vi "FTW-ActorTemplate.vi"(0 "FTW Actor Instance Configuration":string="{\n  \"Identity\": \"ActorName\",\n  \"InboxAddress\": \"tcp://127.0.0.1:*\",\n  \"DebugEnableInboxLogging\": false,\n  \"DebugEnableJobLogging\": false,\n  \"DebugShowPanel\": false\n}", 11 "ErrorIn":errorcluster) -> (15 "Error":errorcluster)   [LabVIEW 2014]
uses:
  src/core/actor/instance/FTW-Actor-Instance.lvclass
  src/core/actor/instance/FTW-Actor-Instance.lvclass/FTW-Actor-Instance.ctl
  src/core/actor/scheduler/FTW-Scheduler-GetNextJob.vi
  src/core/actor/scheduler/FTW-Scheduler-Current.vi
  src/core/actor/request/FTW-Request.lvclass
panel:
  # "Inputs"
  # "Outputs"
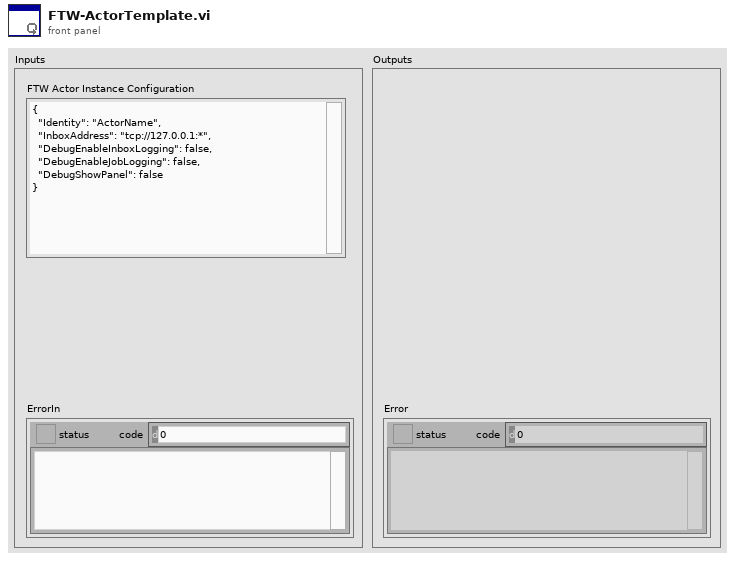
[diagram p1: front panel]
types:
  T1 = cluster{"Incoming Requests":refnum<event-registration>, "Additional Registration Types":refnum<event-registration>}
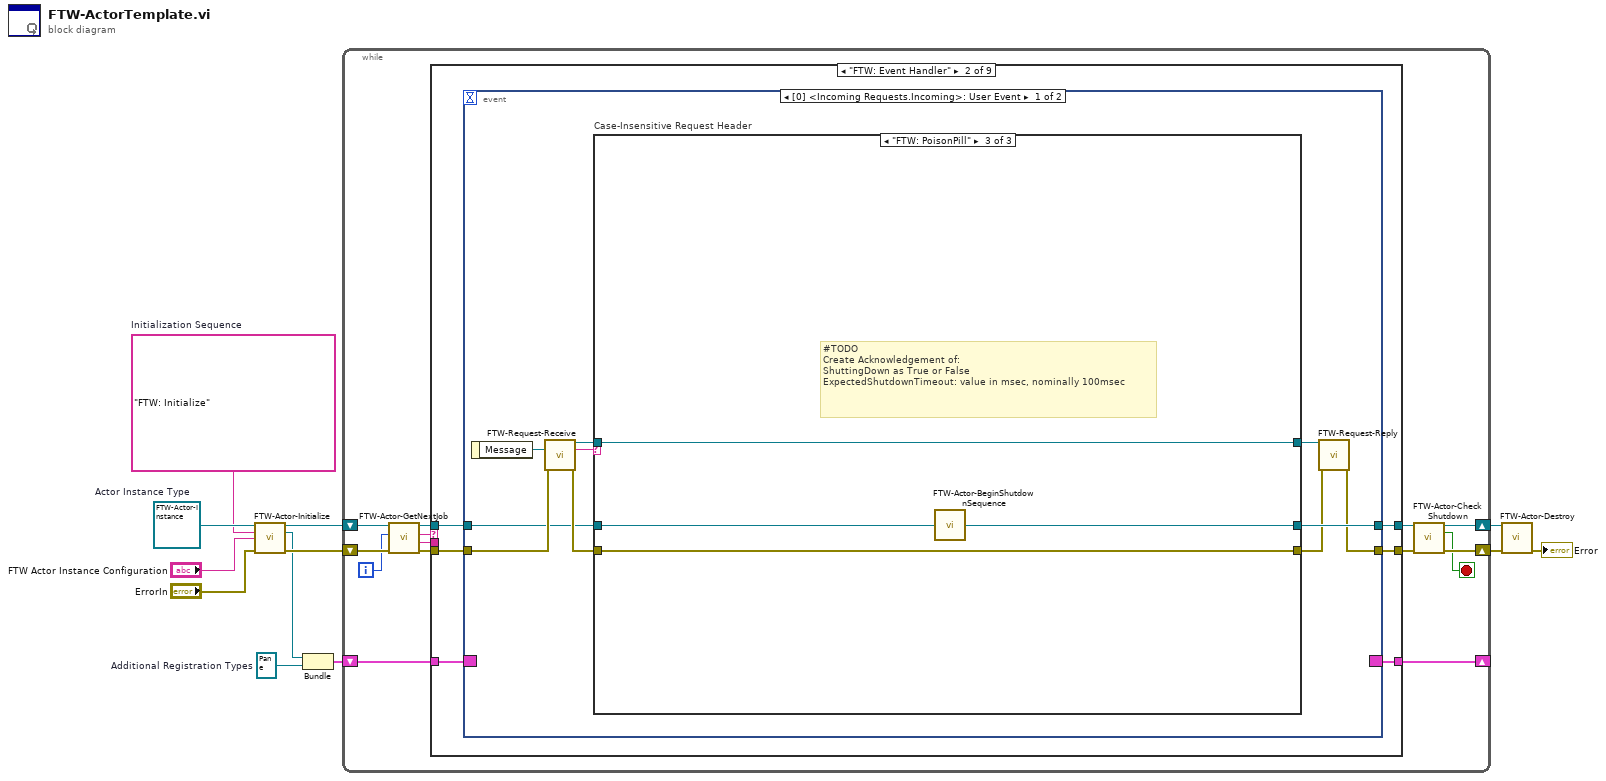
[diagram p0: block diagram]
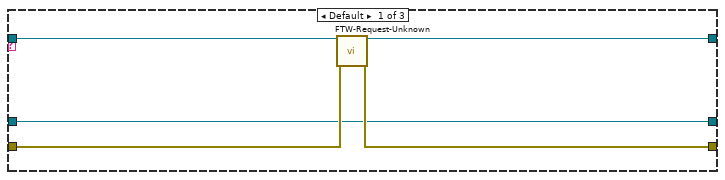
[diagram p3: hidden frame]
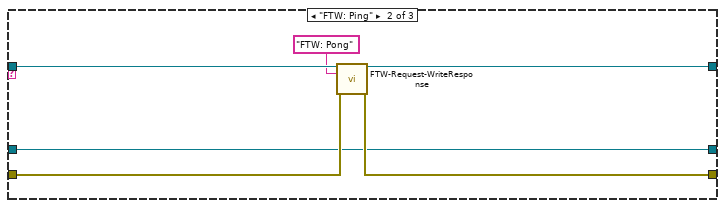
[diagram p4: hidden frame]
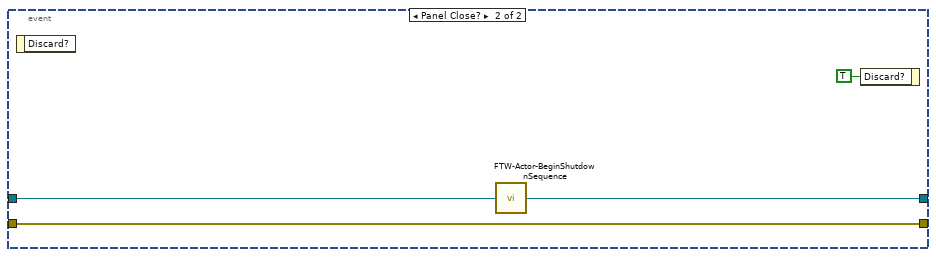
[diagram p5: hidden frame]
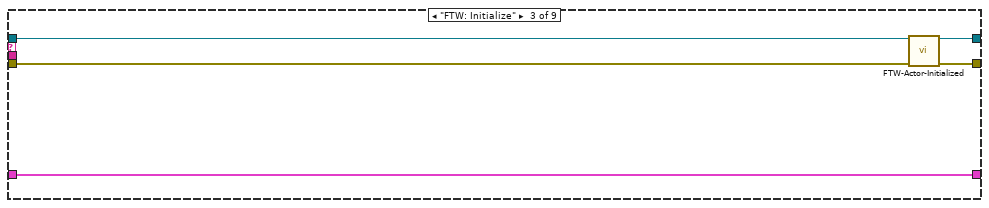
[diagram p6: hidden frame]
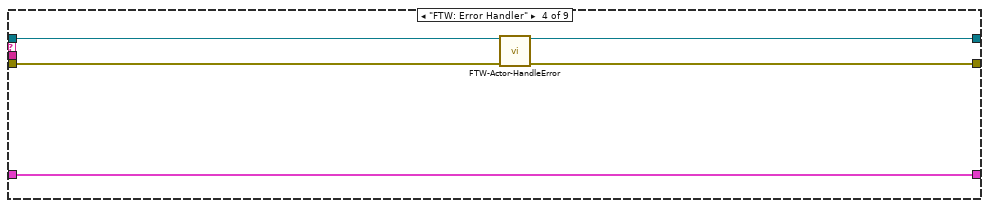
[diagram p7: hidden frame]
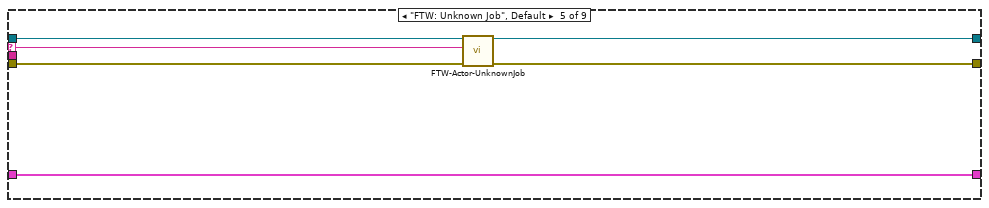
[diagram p8: hidden frame]
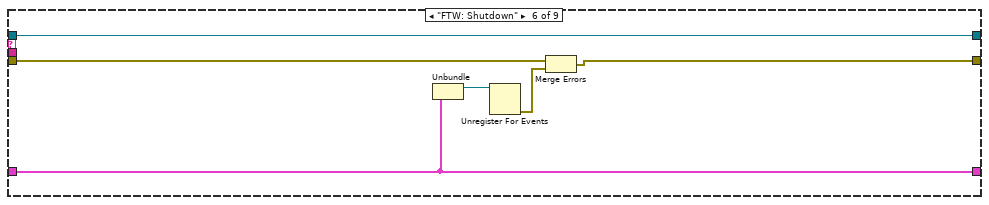
[diagram p9: hidden frame]
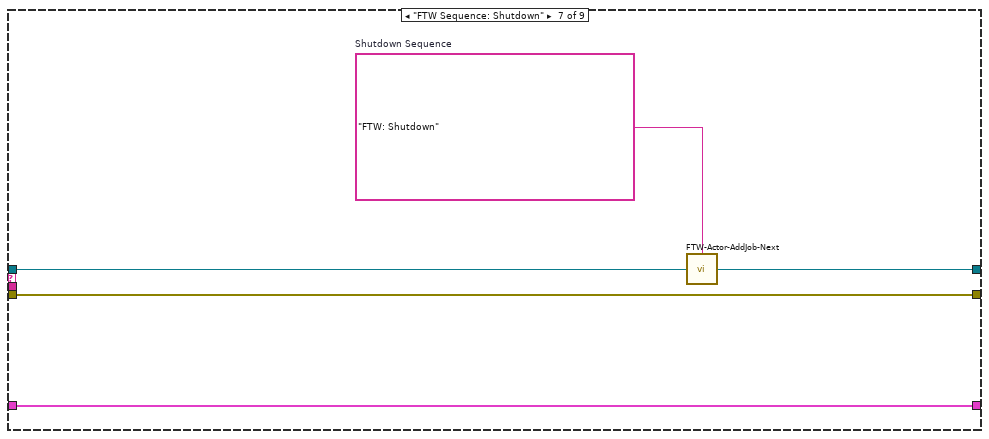
[diagram p10: hidden frame]
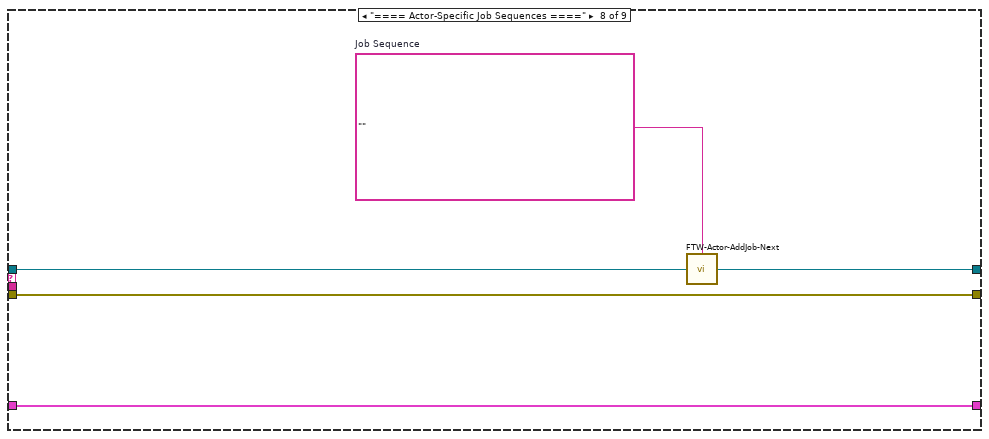
[diagram p11: hidden frame]
diagram:
  w4 = refnum<event-registration> refnum  # Additional Registration Types
  w7 = refnum<class "FTW-Actor-Instance.lvclass"> refnum  # Actor Instance Type
  w6 = "FTW: Initialize"  # Initialization Sequence
  n1 = call "FTW-Actor-Initialize.vi"("FTW Actor Instance Type"=w7, "Initialization Job Sequence"=w6, "Actor Instance Configuration"="FTW Actor Instance Configuration", "error in"="ErrorIn") -> ("FTW Actor Instance"=w12:refnum<class "FTW-Actor-Instance.lvclass">, "Incoming Requests"=w1:refnum<event-registration>, "error out"=w8:errorcluster)  [unwired: 9 in]
  n2 = Bundle("Incoming Requests"=w1, "Additional Registration Types"=w4) -> (w3:T1)  [unwired: 1 in]
  n3 = while {
    shift-right: [w16] -> w10
    shift-left: w8 -> [w23]
    shift-right: [w13] -> _
    shift-left: w3 -> [w26]
    shift-right: [w18] -> w11
    shift-left: w12 -> [w25]
    i -> [w14]
    stop <- w15 stop-if-true
    n4 = call "FTW-Actor-GetNextJob.vi"("error in"=w23, "Jobs Performed"=w14, "FTW Actor Instance"=w25) -> ("error out"=w22:errorcluster, "Job Data"=w20:string, "Job Name"=w21:string, "FTW Actor Instance out"=w24:refnum<class "FTW-Actor-Instance.lvclass">)  [unwired: 5 in]
    n5 = case shown="\"FTW: Event Handler\"" w21 {
      selector: w21 -> [_ _ _ _ w75 _ _ _ _]
      tunnel: [w28 w35 w65 w70 w78 w83 w90 w95 w99] -> w17
      tunnel: w22 -> [w28 w34 w68 w72 w79 w84 w90 w95 w99]
      tunnel: w26 -> [w29 w30 w69 w74 w80 w86 w91 w96 w98]
      tunnel: [w29 w33 w69 w74 w80 w86 w91 w96 w98] -> w13
      tunnel: w20 -> [_ _ _ _ _ _ _ _ _]
      tunnel: [w27 w32 w66 w71 w76 w81 w88 w93 w97] -> w19
      tunnel: w24 -> [w27 w31 w67 w73 w77 w81 w89 w94 w97]
      frame "==== Featherweight Framework Jobs ====" {
      }
      frame "FTW: Event Handler" {
        n6 = event shown="[0] <Incoming Requests.Incoming>: User Event" {
          selector: w30 -> [_ _]
          dyn-events: [_ _] -> w33
          timeout: _ -> [_ _]
          tunnel: [w39 w63] -> w35
          tunnel: w34 -> [w44 w63]
          tunnel: [w43 w61] -> w32
          tunnel: w31 -> [w42 w62]
          event User Event {
            n7 = event-data() -> ("Message"=w36:refnum<class "FTW-Message.lvclass">)  [unwired: 1 in]
            n8 = call "FTW-Request-Receive.vi"("Message"=w36, "error in"=w44) -> ("Initialized Request"=w40:refnum<class "FTW-Request.lvclass">, "Request Header"=w41:string, "error out"=w45:errorcluster)  [unwired: 11 in]
            n9 = case "Case-Insensitive Request Header" shown="\"FTW: PoisonPill\"" w41 {
              tunnel: [w49 w54 w57] -> w38
              tunnel: w45 -> [w50 w55 w57]
              tunnel: [w47 w52 w60] -> w43
              tunnel: w42 -> [w47 w52 w59]
              tunnel: w40 -> [w48 w56 w58]
              tunnel: [w46 w51 w58] -> w37
              frame Default {
                n10 = call "FTW-Request-Unknown.vi"("FTW Incoming Request"=w48, "error in"=w50) -> ("FTW Incoming Request out"=w46:refnum<class "FTW-Request.lvclass">, "error out"=w49:errorcluster)  [unwired: 12 in]
              }
              frame "FTW: Ping" {
                n11 = call "FTW-Request-WriteResponse.vi"("FTW Incoming Request"=w56, "Response Body"="FTW: Pong" ("Response Header"), "error in"=w55) -> ("FTW Incoming Request out"=w51:refnum<class "FTW-Request.lvclass">, "error out"=w54:errorcluster)  [unwired: 11 in]
              }
              frame "FTW: PoisonPill" {
                # "#TODO\nCreate Acknowledgement of:\nShuttingDown as True or False\nExpectedShutdownTimeout: value in msec, nominally 100msec"
                n12 = call "FTW-Actor-BeginShutdownSequence.vi"("FTW Actor Instance"=w59) -> ("FTW Actor Instance out"=w60:refnum<class "FTW-Actor-Instance.lvclass">)  [unwired: 3 in]
              }
            }
            n13 = call "FTW-Request-Reply.vi"("FTW Incoming Request"=w37, "error in"=w38) -> ("error out"=w39:errorcluster)  [unwired: 12 in, 1 out]
          }
          event Panel Close? {
            n14 = event-data() -> ()  [unwired: 1 in, 1 out]
            n15 = call "FTW-Actor-BeginShutdownSequence.vi"("FTW Actor Instance"=w62) -> ("FTW Actor Instance out"=w61:refnum<class "FTW-Actor-Instance.lvclass">)  [unwired: 3 in]
            n16 = event-data("Discard?"=TRUE) -> ()  [unwired: 1 in, 1 out]
          }
        }
      }
      frame "FTW: Initialize" {
        n17 = call-dynamic "FTW-Actor-Initialized.vi"("FTW Actor Instance"=w67, "error in"=w68) -> ("FTW Actor Instance out"=w66:refnum<class "FTW-Actor-Instance.lvclass">, "error out"=w65:errorcluster)  [unwired: 11 in, 1 out]
      }
      frame "FTW: Error Handler" {
        n18 = call-dynamic "FTW-Actor-HandleError.vi"("FTW Actor Instance"=w73, "error in"=w72) -> ("FTW Actor Instance out"=w71:refnum<class "FTW-Actor-Instance.lvclass">, "error out"=w70:errorcluster)  [unwired: 11 in, 1 out]
      }
      frame "FTW: Unknown Job", Default {
        n19 = call-dynamic "FTW-Actor-UnknownJob.vi"("FTW Actor Instance"=w77, "Unknown Job"=w75, "error in"=w79) -> ("FTW Actor Instance out"=w76:refnum<class "FTW-Actor-Instance.lvclass">, "error out"=w78:errorcluster)  [unwired: 11 in]
      }
      frame "FTW: Shutdown" {
        n20 = Unbundle(w86) -> ("Incoming Requests"=w85:refnum<event-registration>)  [unwired: 1 out]
        n21 = Unregister For Events(event registration refnum=w85) -> (error out=w82:errorcluster)  [unwired: 1 in]
        n22 = Merge Errors(w84, w82) -> (w83:errorcluster)
      }
      frame "FTW Sequence: Shutdown" {
        w87 = "FTW: Shutdown"  # Shutdown Sequence
        n23 = call "FTW-Actor-AddJob-Next.vi"("Add Next in Job Queue"=w87, "FTW Actor Instance"=w89) -> ("FTW Actor Instance out"=w88:refnum<class "FTW-Actor-Instance.lvclass">)  [unwired: 2 in]
      }
      frame "==== Actor-Specific Job Sequences ====" {
        w92 = ""  # Job Sequence
        n24 = call "FTW-Actor-AddJob-Next.vi"("Add Next in Job Queue"=w92, "FTW Actor Instance"=w94) -> ("FTW Actor Instance out"=w93:refnum<class "FTW-Actor-Instance.lvclass">)  [unwired: 2 in]
      }
      frame "==== Actor-Specific Jobs ====" {
      }
    }
    n25 = call "FTW-Actor-CheckShutdown.vi"("FTW Actor Instance"=w19, "error in"=w17) -> ("FTW Actor Instance out"=w18:refnum<class "FTW-Actor-Instance.lvclass">, "Shutdown?"=w15:bool, "error out"=w16:errorcluster)  [unwired: 11 in]
  }
  n26 = call-dynamic "FTW-Actor-Destroy.vi"("FTW Actor Instance"=w11, "error in"=w10) -> ("error out"=→"Error":errorcluster)  [unwired: 13 in]
